vi "HandshakeResponse.vi"(6 "additional headers (none)":T1[](array[typedef]), 8 "error in (no error)":errorcluster, 11 "Sec-WebSocket-Key":string) -> (0 "error out":errorcluster, 3 "Response Headers":string)   [LabVIEW 2013, in "WebSockets.lvlib"]
doc: "Creates the HTTP handshaking response."
uses:
  WebSockets.lvlib
  Headers.ctl
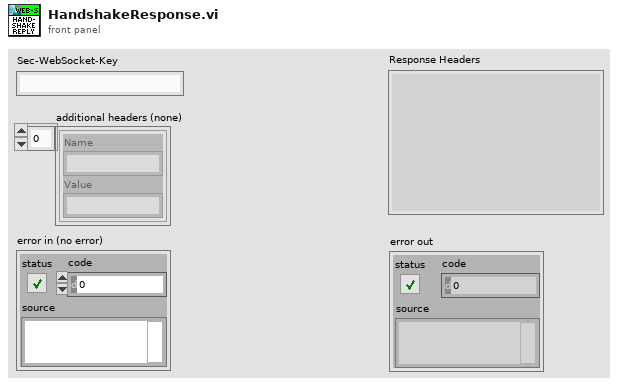
[diagram p1: front panel]
types:
  T1 = typedef "WebSockets.lvlib/Headers.ctl" = cluster{"Name":string, "Value":string}
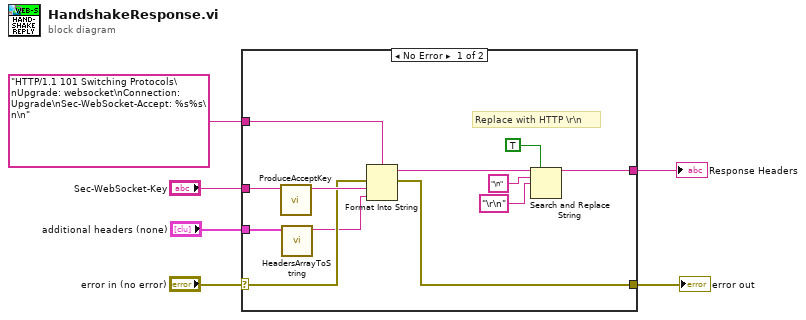
[diagram p0: block diagram]
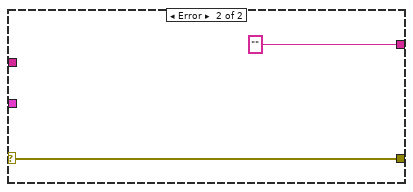
[diagram p2: hidden frame]
diagram:
  n1 = case shown="No Error" "error in (no error)" {
    selector: "error in (no error)" -> [w14 w20]
    tunnel: "Sec-WebSocket-Key" -> [w18 _]
    tunnel: "HTTP/1.1 101 Switching Protocols\nUpgrade: websocket\nConnection: Upgrade\nSec-WebSocket-Accept: %s%s\n\n" ("format string") -> [w17 _]
    tunnel: [w9 ""] -> w5
    tunnel: [w15 w20] -> w3
    tunnel: "additional headers (none)" -> [w7 _]
    frame No Error {
      # "Replace with HTTP \\r\\n"
      n2 = call "ProduceAcceptKey.vi"("Sec-WebSocket-Key"=w18) -> ("Sec-WebSocket-Accept"=w16:string)  [unwired: 10 in]
      n3 = call "HeadersArrayToString.vi"("additional headers (none)"=w7) -> ("header string out"=w8:string)  [unwired: 10 in]
      n4 = Format Into String(format string=w17, error in=w14, w16, w8) -> (resulting string=w10:string, error out=w15:errorcluster)  [unwired: 1 in]
      n5 = Search and Replace String(replace all?=TRUE ("replace all? (F)"), input string=w10, search string="\n" ("search string/char (-)"), replace string="\r\n" ("search string/char (-)")) -> (result string=w9:string)  [unwired: 4 in, 3 out]
    }
    frame Error {
    }
  }
  "Response Headers" <- w5
  "error out" <- w3
